vi "Motic Get Binning Type.vi"(8 "error in (no error)":errorcluster, 11 "camera":i32) -> (0 "error out":errorcluster, 2 "binning type out":u32(ring) items=["Normal", "Sampling", "Fast display"], 3 "camera out":i32)   [LabVIEW 2012, in "MoticApi.lvlib"]
doc: "MOTICAPI bool Motic_getBinningType(MUCam_Handle camera, MUCam_Binning_Type *tl);"
uses:
  MoticApi.lvlib
  MoticApi.dll
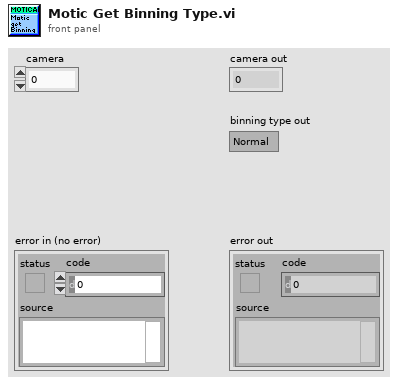
[diagram p1: front panel]
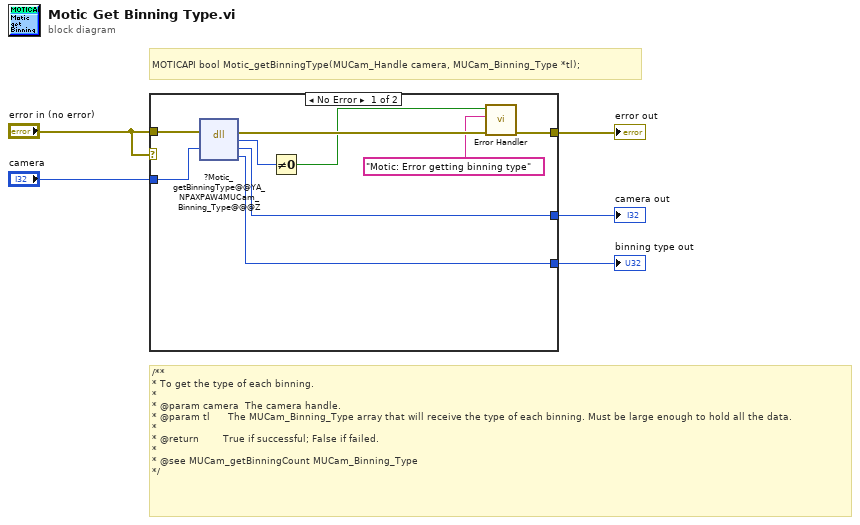
[diagram p0: block diagram]
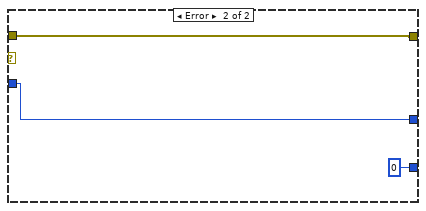
[diagram p2: hidden frame]
diagram:
  # "/**\n* To get the type of each binning.\n*\n* @param camera  The camera handle.\n* @param tl      The MUCam_Binning_Type array that will receive the type of each binning. Must be large enough to hold all the data.\n*\n* @return        True if successful; False if failed.\n*\n* @see MUCam_getBinningCount MUCam_Binning_Type\n*/"
  # "MOTICAPI bool Motic_getBinningType(MUCam_Handle camera, MUCam_Binning_Type *tl);"
  n1 = case shown="No Error" "error in (no error)" {
    tunnel: "camera" -> [w13 w17]
    tunnel: [w12 w17] -> w4
    tunnel: [w11 u32 0 ("tl")] -> w3
    tunnel: "error in (no error)" -> [w10 w16]
    tunnel: [w6 w16] -> w2
    frame No Error {
      n2 = dll-call lib="C:/Users/TTS-Digital/Desktop/MoticApi/MoticApi_git/MoticApi/MoticApi.*" fn="?Motic_getBinningType@@YA_NPAXPAW4MUCam_Binning_Type@@@Z"(error in=w10, "camera"=w13) -> (error out=w9:errorcluster, w14:u8, "camera"=w12:i32, "tl"=w11:u32)  [unwired: 3 in, 1 out]
      n3 = Not Equal To 0?(x=w14) -> (x != 0?=w7:bool)
      n4 = call "Error Handler.vi"("error in (no error)"=w9, "Error message"="Motic: Error getting binning type" ("error message (\"\")"), "Function return"=w7) -> ("error out"=w6:errorcluster)  [unwired: 8 in]
    }
    frame Error {
    }
  }
  "camera out" <- w4
  "binning type out" <- w3
  "error out" <- w2
